vi "InputBitAssignments.vi"(0 "System":u16(ring) items=["Cusp", "Positron", "Musashi"]) -> ()   [LabVIEW 2018]
panel:
  in  "Close (enter)":bool
  out "message":string="Input Bit Assignments\n-----------------------\n00 Sync accumulator\n01 e-source stable"
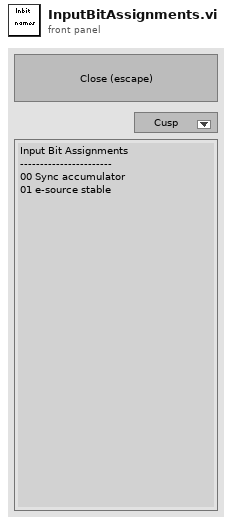
[diagram p1: front panel]
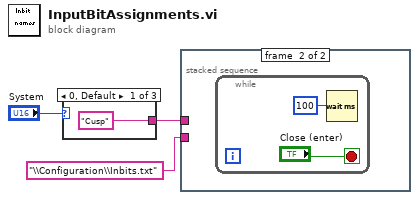
[diagram p0: block diagram]
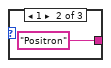
[diagram p2: hidden frame]
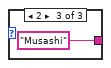
[diagram p3: hidden frame]
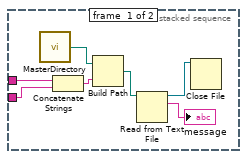
[diagram p4: hidden frame]
diagram:
  n1 = case shown="0, Default" "System" {
    tunnel: ["Cusp" ("string") "Positron" ("string") "Musashi" ("string")] -> w2
    frame 0, Default {
    }
    frame 1 {
    }
    frame 2 {
    }
  }
  n2 = stacked-sequence {
    tunnel: w2 -> [w11 _]
    tunnel: "\\Configuration\\Inbits.txt" ("string") -> [w7 _]
    frame #0 {
      n3 = call "MasterDirectory.vi"() -> ("Master Directory"=w10:path)
      n4 = Concatenate Strings(w11, w7) -> (w9:string)
      n5 = Build Path(base path=w10, name or relative path=w9) -> (appended path=w8:path)
      n6 = Read from Text File(file (use dialog)=w8) -> (refnum out=w12:refnum<file>, text=→"message":string)  [unwired: 3 in, 2 out]
      n7 = Close File(refnum=w12) -> ()  [unwired: 1 in, 2 out]
    }
    frame #1 {
      n8 = while {
        stop <- "Close (enter)" stop-if-true
        n9 = Wait (ms)(milliseconds to wait=u32 100) -> ()  [unwired: 1 out]
      }
    }
  }
